vi "ConfigureCurrent.vi"(8 "error in (no error)":errorcluster, 10 "Current(0)":dbl, 11 "YP03-60_X in":refnum<class "YP03-60_X.lvclass">) -> (0 "error out 2":errorcluster, 3 "YP03-60_X out":refnum<class "YP03-60_X.lvclass">)   [LabVIEW 2020, in "PowerControl.lvlib" / "YP03-60_X.lvclass"]
uses:
  YP03-60_X.lvclass
  YP03-60_X.lvclass/YP03-60_X.ctl
  <vilib>/Instr/_visa.llb/VISA Configure Serial Port (Instr).vi
  VirtualPower/VirtualPower.lvclass
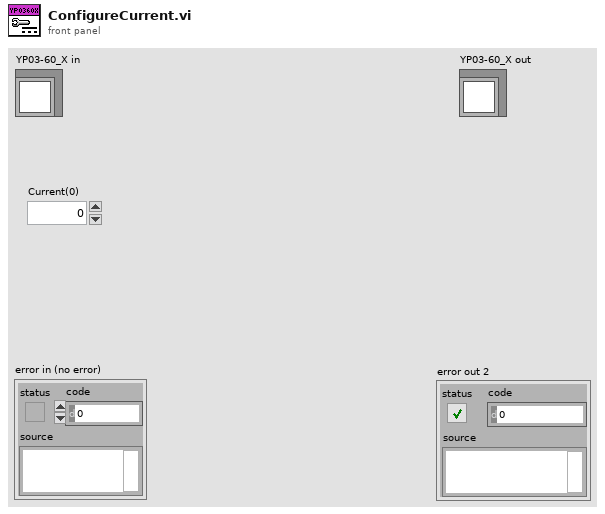
[diagram p1: front panel]
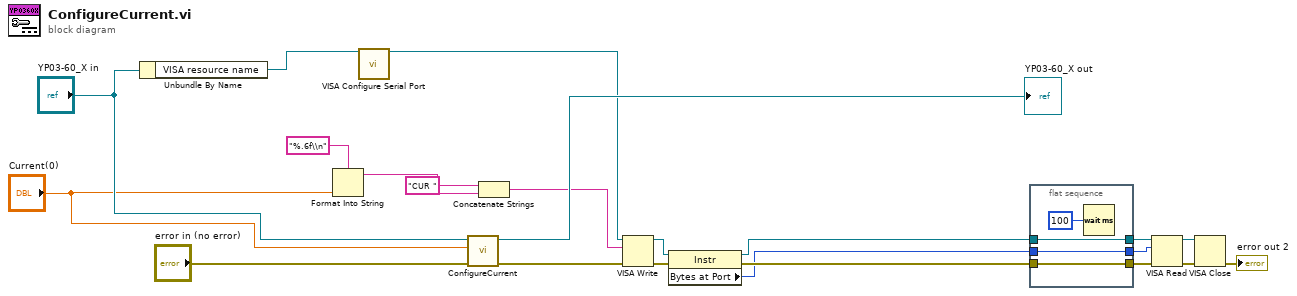
[diagram p0: block diagram]
diagram:
  n1 = Unbundle By Name("YP03-60_X in") -> ("VISA resource name"=w5:refnum<visa-resource-name>)
  n2 = Format Into String(format string="%.6f\\n", "Current(0)") -> (resulting string=w14:string)  [unwired: 2 in, 1 out]
  n3 = call-poly "VISA Configure Serial Port"("VISA resource name"=w5) -> ("VISA resource name out"=w4:refnum<visa-resource-name>)  [unwired: 13 in, 1 out]
  n4 = call-parent "ConfigureCurrent.vi"("error in (no error)"="error in (no error)", "Current(0)"="Current(0)", "VirtualPower in"="YP03-60_X in") -> ("error out"=w10:errorcluster, "VirtualPower out"=→"YP03-60_X out":refnum<class "YP03-60_X.lvclass">)  [unwired: 7 in]
  n5 = Concatenate Strings("CUR " ("string"), w14) -> (w11:string)
  n6 = VISA Write(VISA resource name=w4, write buffer=w11, error in (no error)=w10) -> (VISA resource name out=w9:refnum<visa-resource-name>, error out=w8:errorcluster)  [unwired: 1 out]
  n7 = property class="Instr"(reference=w9, error in=w8) -> (reference out=w17:refnum<visa-resource-name>, error out=w19:errorcluster, "Bytes at Port"=w15:u32)
  n8 = flat-sequence {
    tunnel: w17 -> [w26]
    tunnel: [w26] -> w18
    tunnel: [w25] -> w20
    tunnel: w19 -> [w25]
    tunnel: [w24] -> w16
    tunnel: w15 -> [w24]
    frame #0 {
      n9 = Wait (ms)(milliseconds to wait=u32 100) -> ()  [unwired: 1 out]
    }
  }
  n10 = VISA Read(VISA resource name=w18, byte count=w16, error in (no error)=w20) -> (VISA resource name out=w3:refnum<visa-resource-name>, error out=w1:errorcluster)  [unwired: 2 out]
  n11 = VISA Close(VISA resource name=w3, error in (no error)=w1) -> (error out=→"error out 2":errorcluster)
